vi "FPGA_decipher_order.vi"(11 "order in":u64) -> (0 "data 1":u8, 1 "data 2":u8, 2 "data 3":u8, 3 "data 4":u8, 4 "RFU 2":u8, 5 "order out":u8, 6 "RFU 1":u8, 7 "subsystem":u8)   [LabVIEW 2013]
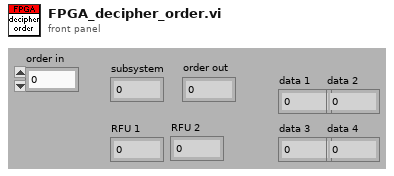
[diagram p1: front panel]
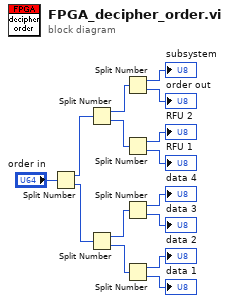
[diagram p0: block diagram]
diagram:
  n1 = Split Number(x="order in") -> (hi(x)=w14:u32, lo(x)=w15:u32)
  n2 = Split Number(x=w14) -> (hi(x)=w10:u16, lo(x)=w11:u16)
  n3 = Split Number(x=w15) -> (hi(x)=w12:u16, lo(x)=w13:u16)
  n4 = Split Number(x=w10) -> (hi(x)=→"subsystem":u8, lo(x)=→"order out":u8)
  n5 = Split Number(x=w11) -> (hi(x)=→"RFU 2":u8, lo(x)=→"RFU 1":u8)
  n6 = Split Number(x=w12) -> (hi(x)=→"data 4":u8, lo(x)=→"data 3":u8)
  n7 = Split Number(x=w13) -> (hi(x)=→"data 2":u8, lo(x)=→"data 1":u8)
